vi "To Generic.vi"(8 "error in (no error)":errorcluster, 11 "Instrument Error Data in":refnum<class "Instrument List Data.lvclass">) -> (0 "error out":errorcluster, 2 "Generic Data":refnum<class "Generic Data.lvclass">[](array[class]), 3 "Data Name":string[](array[string]))   [LabVIEW 2020, in "Instrument Handler.lvlib" / "Instrument List Data.lvclass"]
doc: "Present private data as an array of named generic data elements."
uses:
  Instrument List Data.lvclass
  PPL/HDH.Data.Generic.lvlibp/Generic Data/Generic Data.lvclass
  Instrument List Data.lvclass/Instrument List Data.ctl
  PPL/HDH.Data.Generic.lvlibp/Generic Data/Generic Array Data/Boolean Array/Boolean Array.lvclass
  C:/Current projects/WS/PPL/HDH.Data.Generic.lvlibp/Generic Data/Generic Array Data/Generic Array Data.lvclass
  PPL/HDH.Data.Generic.lvlibp/Generic Data/Generic Array Data/U32 Array/U32 Array.lvclass
  PPL/HDH.Data.Generic.lvlibp/Generic Data/Generic Array Data/String Array/String Array.lvclass
  PPL/HDH.Data.Generic.lvlibp/Generic Data/Generic Array Data/Generic Array Data.lvclass
  C:/Current projects/WS/PPL/HDH.Data.Generic.lvlibp/Generic Data/Generic Data.lvclass
  PPL/HDH.Data.Generic.lvlibp/Data.lvclass
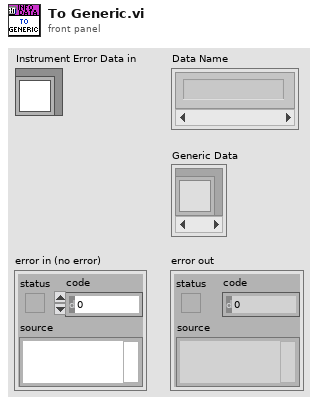
[diagram p1: front panel]
types:
  T1 = typedef "Instrument Handler.lvlib/Ctl_InstrumentInfo.ctl" = cluster{"Launched?":bool, "Instrument ID":u32, "Driver":string, "Alias":string, "Connection Type":string}
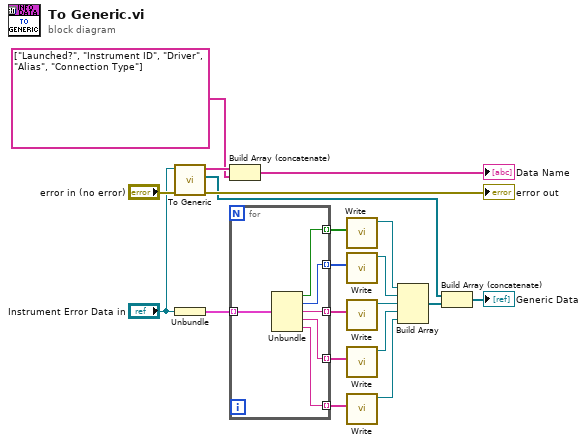
[diagram p0: block diagram]
diagram:
  n1 = call-parent "To Generic.vi"("error in (no error)"="error in (no error)", "Data in"="Instrument Error Data in") -> ("error out"=→"error out":errorcluster, "Generic Data"=w14:refnum<class "Generic Data.lvclass">[], "Data Name"=w17:string[])  [unwired: 7 in]
  n2 = Unbundle("Instrument Error Data in") -> (w12:T1[])
  n3 = Build Array (concatenate)(w17, string[] ["Launched?", "Instrument ID", "Driver", "Alias", "Connection Type"] ("array")) -> (→"Data Name":string[])
  n4 = for {
    tunnel: w12 -> [w26] mode=indexing
    tunnel: [w25] -> w11 mode=indexing
    tunnel: [w22] -> w8 mode=indexing
    tunnel: [w23] -> w6 mode=indexing
    tunnel: [w24] -> w4 mode=indexing
    tunnel: [w21] -> w2 mode=indexing
    n5 = Unbundle(w26) -> ("Launched?"=w25:bool, "Instrument ID"=w21:u32, "Driver"=w22:string, "Alias"=w23:string, "Connection Type"=w24:string)
  }
  n6 = call "Write.vi"("Boolean Array"=w11) -> ("Boolean Array out"=w10:refnum<class "Boolean Array.lvclass">)  [unwired: 10 in]
  n7 = call "Write.vi"("U32 Array"=w2) -> ("U32 Array out"=w1:refnum<class "U32 Array.lvclass">)  [unwired: 10 in]
  n8 = call "Write.vi"("String Array"=w8) -> ("String Array out"=w7:refnum<class "String Array.lvclass">)  [unwired: 10 in]
  n9 = call "Write.vi"("String Array"=w6) -> ("String Array out"=w5:refnum<class "String Array.lvclass">)  [unwired: 10 in]
  n10 = call "Write.vi"("String Array"=w4) -> ("String Array out"=w3:refnum<class "String Array.lvclass">)  [unwired: 10 in]
  n11 = Build Array(w10, w1, w7, w5, w3) -> (w9:refnum<class "Generic Array Data.lvclass">[])
  n12 = Build Array (concatenate)(w14, w9) -> (→"Generic Data":refnum<class "Generic Data.lvclass">[])
